vi "Basic_HVOF_Run.vi"   [LabVIEW 2018]
uses:
  Global Variables.vi
types:
  T1 = enum32{"Invalid", "Standard", "Closed", "Hidden", "Minimized", "Maximized"}
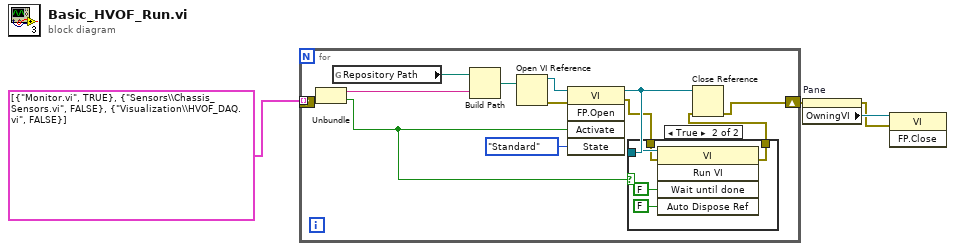
[diagram p0: block diagram]
diagram:
  n1 = for {
    tunnel: cluster{string, bool}[] [{"Monitor.vi", TRUE}, {"Sensors\\Chassis_Sensors.vi", FALSE}, {"Visualization\\HVOF_DAQ.vi", FALSE}] -> [w15] mode=indexing
    shift-right: [w10] -> w4
    shift-left: _ -> [_]
    n2 = Unbundle(w15) -> (w9:string, w7:bool)
    n3 = global read "Global Variables.vi" "Repository Path"() -> (w16:path)
    n4 = Build Path(base path=w16, name or relative path=w9) -> (appended path=w14:path)
    n5 = Open VI Reference(vi path=w14) -> (vi reference=w13:refnum<vi>, error out=w12:errorcluster)  [unwired: 5 in]
    n6 = invoke class="VI" method="FP.Open"(reference=w13, error in=w12, "Activate"=w7, "State"=T1."Standard") -> (reference out=w8:refnum<vi>, error out=w6:errorcluster)  [unwired: 1 in, 3 out]
    n7 = case shown="True" w7 {
      tunnel: w8 -> [_ w22]
      tunnel: w6 -> [w17 w19]
      tunnel: [w17 w18] -> w5
      frame False {
      }
      frame True {
        n8 = invoke class="VI" method="Run VI"(reference=w22, error in=w19, "Wait until done"=FALSE ("Wait Until Done"), "Auto Dispose Ref"=FALSE ("Auto Dispose Reference")) -> (error out=w18:errorcluster)  [unwired: 1 in, 4 out]
      }
    }
    n9 = Close Reference(reference=w8, error in (no error)=w5) -> (error out=w10:errorcluster)
  }
  n10 = property on="Pane" class="Pane"(error in=w4) -> (error out=w2:errorcluster, "OwningVI"=w3:refnum<vi>)  [unwired: 1 in, 1 out]
  n11 = invoke class="VI" method="FP.Close"(reference=w3, error in=w2) -> ()  [unwired: 1 in, 3 out]
